vi "tx_pduGen.vi"(5 "byte array":u8[](array[numeric])) -> (0 "packet bits length":i32, 2 "pdu":i32[](array[numeric]))   [LabVIEW 2014]
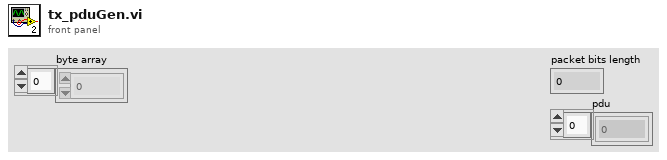
[diagram p1: front panel]
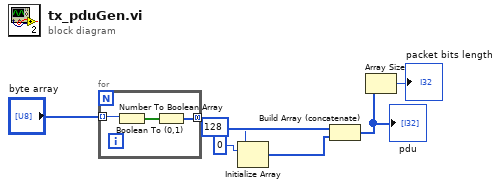
[diagram p0: block diagram]
diagram:
  n1 = for {
    tunnel: "byte array" -> [w10] mode=indexing
    tunnel: [w8] -> w6 mode=concatenating
    n2 = Number To Boolean Array(number=w10) -> (Boolean array=w9:bool[])
    n3 = Boolean To (0,1)(Boolean=w9) -> (0, 1=w8:i16[])
  }
  n4 = Initialize Array(u8 0, 128 ("dimension size")) -> (w1:u8[])
  n5 = Build Array (concatenate)(w6, w1) -> (w5:i16[])
  "pdu" <- w5
  n6 = Array Size(array=w5) -> (size(s)=→"packet bits length":i32)
